vi "SCMP - Externally Triggered Image Acquisition - v3.vi"(0 "FPS":dbl=10.0 format="%.1g", 1 "LCVR Voltages":dbl[][](array[numeric]), 5 "Modulation Cycles":i32=1 min=1 max=30 step=1, 7 "Save to FITS?":bool=TRUE, 9 "Headers In":T12[](array[typedef])=[{"Wavelength (nm)"=530.15, "Exposure (s)"=0.05, "Tuning Delay (ms)"=1000.0, "Beam Type (-1/1)"=1.0, "Tuning Voltages"=[1.111, 2.222, 3.333, 4.444], "Observer"="observer", "Light Shapping Diffuser"=enum."In Beam", "Comment"="", "Data Type"=9, "Mod Cycles"=0, "SCD Calibration Optics"=enum."1 - Polarizer @0, I+Q", "SCD Emission Line Filter"=enum."1-557.6nm", "Cookbook"="", "COMP-S Calibration Wheel"=enum."Dark", "COMP-S Andover Filter Wheel"=enum."530.3nm/HWB 0.34nm (Fe XIV)", "FOV Rotation (deg)"=66.0, "Objective Lens Position (mm)"=0.0, "Occulter size"=0.0, "Time End"=timestamp(3382374145.421875 s since 1904-01-01), "Acc Exposure (s)"=0.0, "Time Stamp Array"=[], "Camera Serial Number"=[], "Camera Temp"=[], "Camera PI (mm)"=[], "Time Start"=timestamp(3382374145.421875 s since 1904-01-01), "Peripherals"={"ILX controler"=FALSE, "Zone temperatures"=FALSE, "Andor"=FALSE, "Andor 2"=FALSE, "PI Stages"=FALSE, "AISAS mechanisms"=FALSE, "AISAS Mech.lvclass"=refnum, "Zone temp ref"=variant, "FWs"=FALSE}, "FITS paths"=[], "Cameras"=enum."Andor", "load preset cbk"=FALSE, "periodic check count"=0, "COMP-S Calibration Wheel 2"=enum."Dark", "Calib"=enum."Dark", "Abso Aperture"=40.0, "Nominal Aperture"=196.0}] {"Nominal Aperture" format="%.1f"; "Abso Aperture" format="%.1f"; "Camera PI (mm)" format="%_3g"; "Acc Exposure (s)" format="%^.3g"; "Occulter size" format="%.2f"; "Objective Lens Position (mm)" min=70.0 max=152.0 format="%.2f"; "FOV Rotation (deg)" format="%.1f"; "Data Type" items=["LIVE", "DARK", "FLAT", "CALI", "OBSE", "ABSO", "AURE", "TARG", "OBJE", "HOLE", "OREX", "THRO", "CHIP"]; "Exposure (s)" format="%^.3g"; "Wavelength (nm)" format="%_6g"}, 11 "error in":errorcluster, 12 "Andor Neo":T13[](array[typedef]) {"Exposure (s)" format="%^.3g"; "Time at Synch" format="%<%H:%M:%S>T"; "Interframe Time" format="%#_3g"; "Frame Readout Time" format="%_3g"; "Row Readout Time" format="%_3g"}) -> (3 "FITS Path Out":path, 6 "Image":u32[][](array[numeric]), 8 "Image Cam2":u32[][](graph), 10 "Headers Out":T2[](array[typedef]) {"Nominal Aperture" format="%.1f"; "Abso Aperture" format="%.1f"; "Camera PI (mm)" format="%_3g"; "Acc Exposure (s)" format="%^.3g"; "Occulter size" format="%.2f"; "Objective Lens Position (mm)" min=70.0 max=152.0 format="%.2f"; "FOV Rotation (deg)" format="%.1f"; "Exposure (s)" format="%^.3g"; "Wavelength (nm)" format="%_6g"}, 13 "FITS Path Out 2":path, 14 "Break":bool, 15 "error out":errorcluster)   [LabVIEW 2014]
doc: "The LL Sequence VI acquires a sequence of images and displays them in an array of image controls using the low-level acquisition VIs. A sequence is appropriate for applications that process multiple images. You can configure a sequence to acquire every frame or to skip a variable number of frames between each image.\n\nTop Level Code Overview\n1) Initialize Camera (Global Shutter, High Well, Low Noise, exposure time, etc.)\n2) Create a buffer set equal in size to the # of trigger pulses (e.g. 100) which is the same as the # of expected images \n3) Start the camera acquisition THEN start the DAQmx task (use merge error cluster to gurantee this)"
uses:
  Camera/Andor Neo Info.ctl
  Controls/run cbk timeout.ctl
  <vilib>/Waveform/WDTOps.llb/WDT Waveform Duration DBL.vi
  <vilib>/DAQmx/write.llb/DAQmx Write (Analog 1D Wfm NChan NSamp).vi
  <vilib>/DAQmx/create/channels.llb/DAQmx Create Channel (AO-Voltage-Basic).vi
  <vilib>/DAQmx/configure/timing.llb/DAQmx Timing (Use Waveform).vi
  Controls/beaning.ctl
  Controls/SCD - Calibration Optics Filter Wheel.ctl
  AISAS/Controls/Diffuser.ctl
  Controls/SCD - FITS Cluster.ctl
  Controls/SCD - EDT - Emission Line Filter Wheel.ctl
  Controls/CoMP-S Controls/Polarization Optics Filter Wheel.ctl
  Controls/CoMP-S Controls/Emission Line Filter Wheel.ctl
  AISAS/Controls/focus.ctl
  AISAS/Mech/AISAS Mech.lvclass
  Controls/peripherals.ctl
  Controls/Cameras select.ctl
  Controls/FITS Data type.ctl
panel:
  out "error dequeue RAM":errorcluster
  out "mod cycles *4":i32=1
  out "error cam dequeue & queue RAM":errorcluster
  out "error dequeue 2":errorcluster
  in  "count 2":i32
  in  "Tab Control":T1(tab)
  out "# elements in RAM queue":i32
  out "Image Acq (s)":dbl(slide)=4151.832132564842
  out "Image display & SSD Saving":i32(slide) scale=0.0..1.0
  in  "user break":bool
  out "Image Cam1 wide":u32[][](graph)
  out "Image Cam1":u32[][](graph)
  out "# images to acquire":i32
  out "Image Acquisition Started":bool
  out "PixelData [U16]":u16[](array[numeric])
  out "ByteData [U8]":u8[](array[numeric])
  in  "image pointers":u64[](array[numeric])
  in  "imageNo":i32
  in  "count":i32
  out "# wavelengths":i32=1
  out "Exposure Get (s)":dbl=0.09 format="%_3p"
  out "# elements in queue":i32
  out "Image Cam":u32[][](graph)
  out "# buffer":i32
  in  "image pointers 2":u64[](array[numeric])
  in  "imageNo 2":i32
  out "# elements in queue 2":i32
  out "# buffer 2":i32
  out "Image transfering":u32(slide) scale=0.0..4.0
  out "Acquisition Estimate (s)":dbl format="%0.2f"
  out "Image Acq":i32(slide) scale=0.0..4.0
  out "Time Start":timestamp=timestamp(3382374145.421875 s since 1904-01-01) format="%<%H:%M:%S%3u\n%x>T"
  out "Time stamp arr":timestamp[](array[timestamp]) format="%<%H:%M:%S%3u>T"
  out "COMP Waveforms":waveform(dbl)[](graph)
  out "SCD Waveforms":waveform(dbl)[](graph)
  out "Time stamp arr 2":timestamp[](array[timestamp]) format="%<%H:%M:%S%3u>T"
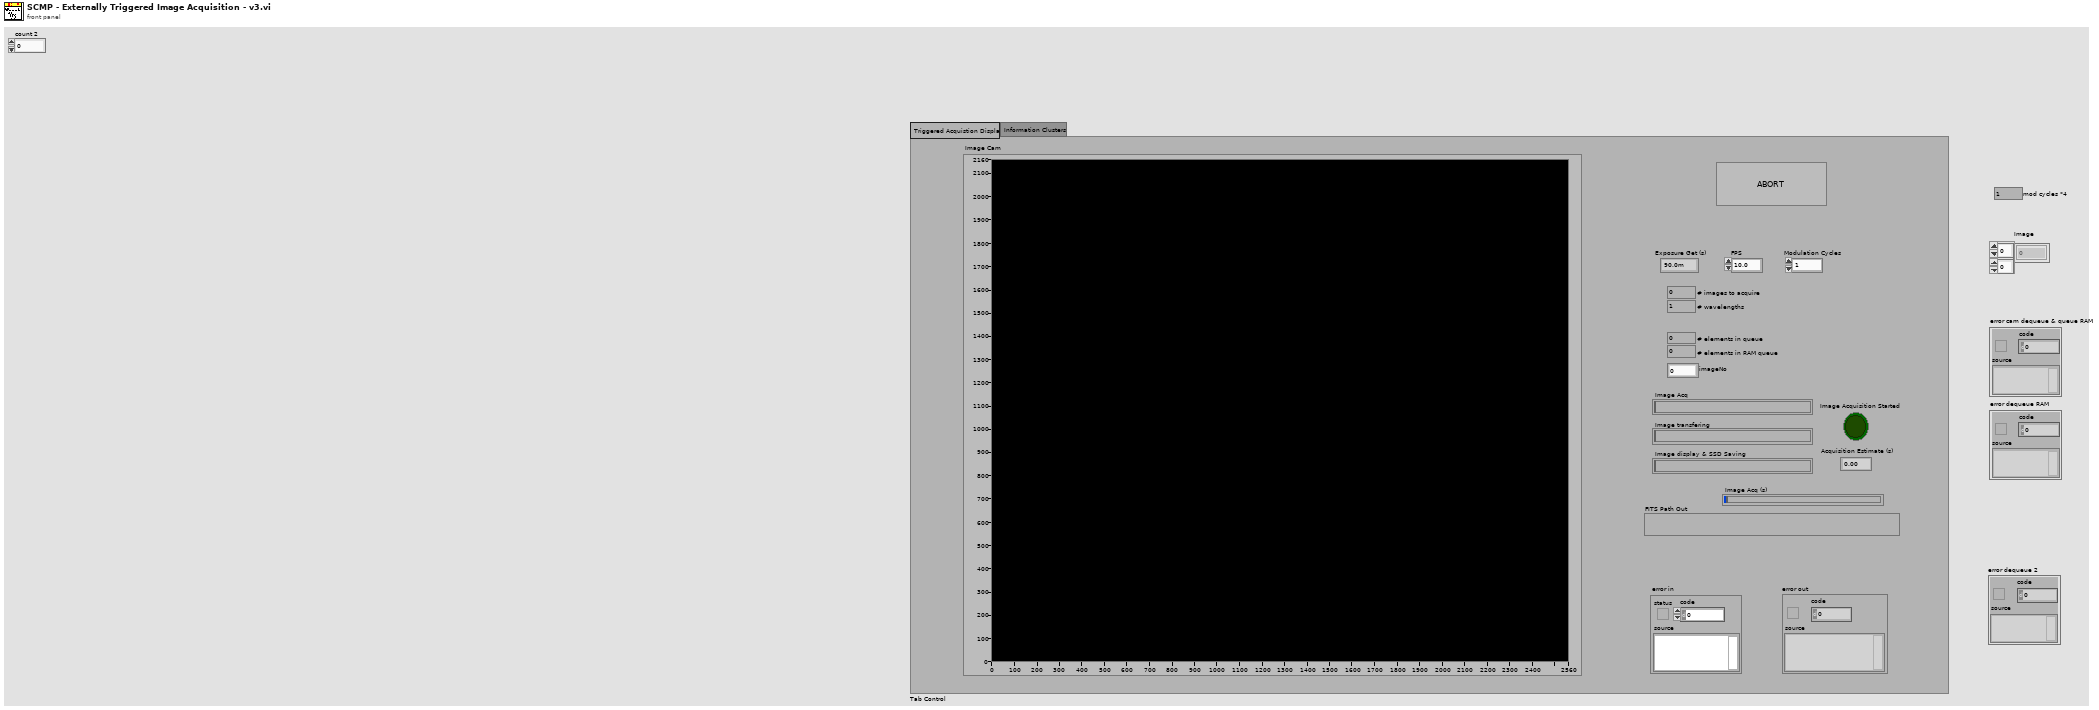
[diagram p1: front panel]
types:
  T1 = enum32{"Triggered Acquistion Display", "Information Clusters"}
  T2 = typedef "SCD - FITS Cluster.ctl" = cluster{"Wavelength (nm)":dbl, "Exposure (s)":dbl, "Tuning Delay (ms)":dbl, "Beam Type (-1/1)":dbl, "Tuning Voltages":dbl[], "Observer":string, "Light Shapping Diffuser":T3, "Comment":string, "Data Type":T4, "Mod Cycles":u16, "SCD Calibration Optics":T5, "SCD Emission Line Filter":T6, "Cookbook":string, "COMP-S Calibration Wheel":T7, "COMP-S Andover Filter Wheel":T8, "FOV Rotation (deg)":dbl, "Objective Lens Position (mm)":T9, "Occulter size":dbl, "Time End":timestamp, "Acc Exposure (s)":dbl, "Time Stamp Array":timestamp[], "Camera Serial Number":string[], "Camera Temp":dbl[], "Camera PI (mm)":dbl[], "Time Start":timestamp, "Peripherals":T10, "FITS paths":path[], "Cameras":T11, "load preset cbk":bool, "periodic check count":i32, "COMP-S Calibration Wheel 2":T7, "Calib":enum16{"Dark", "Flat"}, "Abso Aperture":dbl, "Nominal Aperture":dbl, "Pointer IP":string}
  T3 = typedef "Diffuser.ctl" = enum16{"Out of Beam", "In Beam"}
  T4 = typedef "FITS Data type.ctl" = enum16{"LIVE", "DARK", "FLAT", "CALI", "OBSE", "ABSO", "AURE", "TARG", "OBJE", "HOLE", "OREX", "THRO", "CHIP"}
  T5 = typedef "SCD - Calibration Optics Filter Wheel.ctl" = enum16{"1 - Polarizer @0, I+Q", "2 - Polarizer @90, I-Q", "3 - Polarizer @45, I+U", "4 - Polarizer @135, I-U", "5 - Polarizer @0, Retarder @45, I+V", "6 - Polarizer @0, Retarder @135, I-V", "7 - Dark", "8 - Clear", "9 - N/A"}
  T6 = typedef "SCD - EDT - Emission Line Filter Wheel.ctl" = enum16{"1-557.6nm", "2-587.6nm", "3-589.6nm", "4-630.2nm", "5-656.4nm", "6-849.8nm", "7-854.2nm", "8-866.2nm", "9-1083.0nm"}
  T7 = typedef "Polarization Optics Filter Wheel.ctl" = enum16{"Dark", "Clear", "Exchange Lens", "Polarizer @0, I+Q", "Polarizer @90, I-Q", "Polarizer @45, I+U", "Polarizer @135, I-U", "Polarizer @0, Retarder @45, I+V", "Polarizer @0, Retarder @135, I-V"}
  T8 = typedef "Emission Line Filter Wheel.ctl" = enum16{"530.3nm/HWB 0.34nm (Fe XIV)", "587.6nm/HBW 0.44nm (He I D3)", "637.5nm/HBW 0.53nm (Fe X)", "656.3nm/HBW 0.57nm (H-Alpha)", "789.2nm/HBW 0.85nm (Fe XI)", "854.2nm/HBW 1.01nm (Ca I)", "1074.7nm/HBW 2.34nm (Fe XIII)", "1079.8nm/HBW 1.64nm (Fe XIII)", "1083.0nm/HBW 1.66nm (He I)"}
  T9 = typedef "focus.ctl" = dbl
  T10 = typedef "peripherals.ctl" = cluster{"ILX controler":bool, "Zone temperatures":bool, "Andor":bool, "Andor 2":bool, "PI Stages":bool, "AISAS mechanisms":bool, "AISAS Mech.lvclass":refnum<class "AISAS Mech.lvclass">, "Zone temp ref":variant, "FWs":bool}
  T11 = typedef "Cameras select.ctl" = enum16{"Andor", "GDR"}
  T12 = typedef "SCD - FITS Cluster.ctl" = cluster{"Wavelength (nm)":dbl, "Exposure (s)":dbl, "Tuning Delay (ms)":dbl, "Beam Type (-1/1)":dbl, "Tuning Voltages":dbl[], "Observer":string, "Light Shapping Diffuser":T3, "Comment":string, "Data Type":u16, "Mod Cycles":u16, "SCD Calibration Optics":T5, "SCD Emission Line Filter":T6, "Cookbook":string, "COMP-S Calibration Wheel":T7, "COMP-S Andover Filter Wheel":T8, "FOV Rotation (deg)":dbl, "Objective Lens Position (mm)":T9, "Occulter size":dbl, "Time End":timestamp, "Acc Exposure (s)":dbl, "Time Stamp Array":timestamp[], "Camera Serial Number":string[], "Camera Temp":dbl[], "Camera PI (mm)":dbl[], "Time Start":timestamp, "Peripherals":T10, "FITS paths":path[], "Cameras":T11, "load preset cbk":bool, "periodic check count":i32, "COMP-S Calibration Wheel 2":T7, "Calib":enum16{"Dark", "Flat"}, "Abso Aperture":dbl, "Nominal Aperture":dbl}
  T13 = typedef "Andor Neo Info.ctl" = cluster{"Handle":i32, "Pixel Encoding":string, "AOI Width":i32, "AOI Height":i32, "AOI Stride":i32, "Row Readout Time":dbl, "Frame Readout Time":dbl, "Interframe Time":dbl, "Semaphore":T14, "SerialNumber":string, "Camera Model":string, "Controller ID":string, "Firmware Version":string, "Shutter":string, "BDiv":u8, "Time at Synch":timestamp, "Idx":i32, "PreAmp":string, "Binning":T15, "PixelReadoutRate":string, "Exposure (s)":dbl, "Image Bytes":i64, "Image Pixels":i64, "SpuriousNoiseFilter":bool, "Overlap":bool, "CycleMode":string}
  T14 = typedef "Semaphore RefNum" = refnum<k1>
  T15 = typedef "beaning.ctl" = enum16{"1x1", "2x2", "3x3", "4x4", "8x8"}
  T16 = typedef "run cbk timeout.ctl" = i32
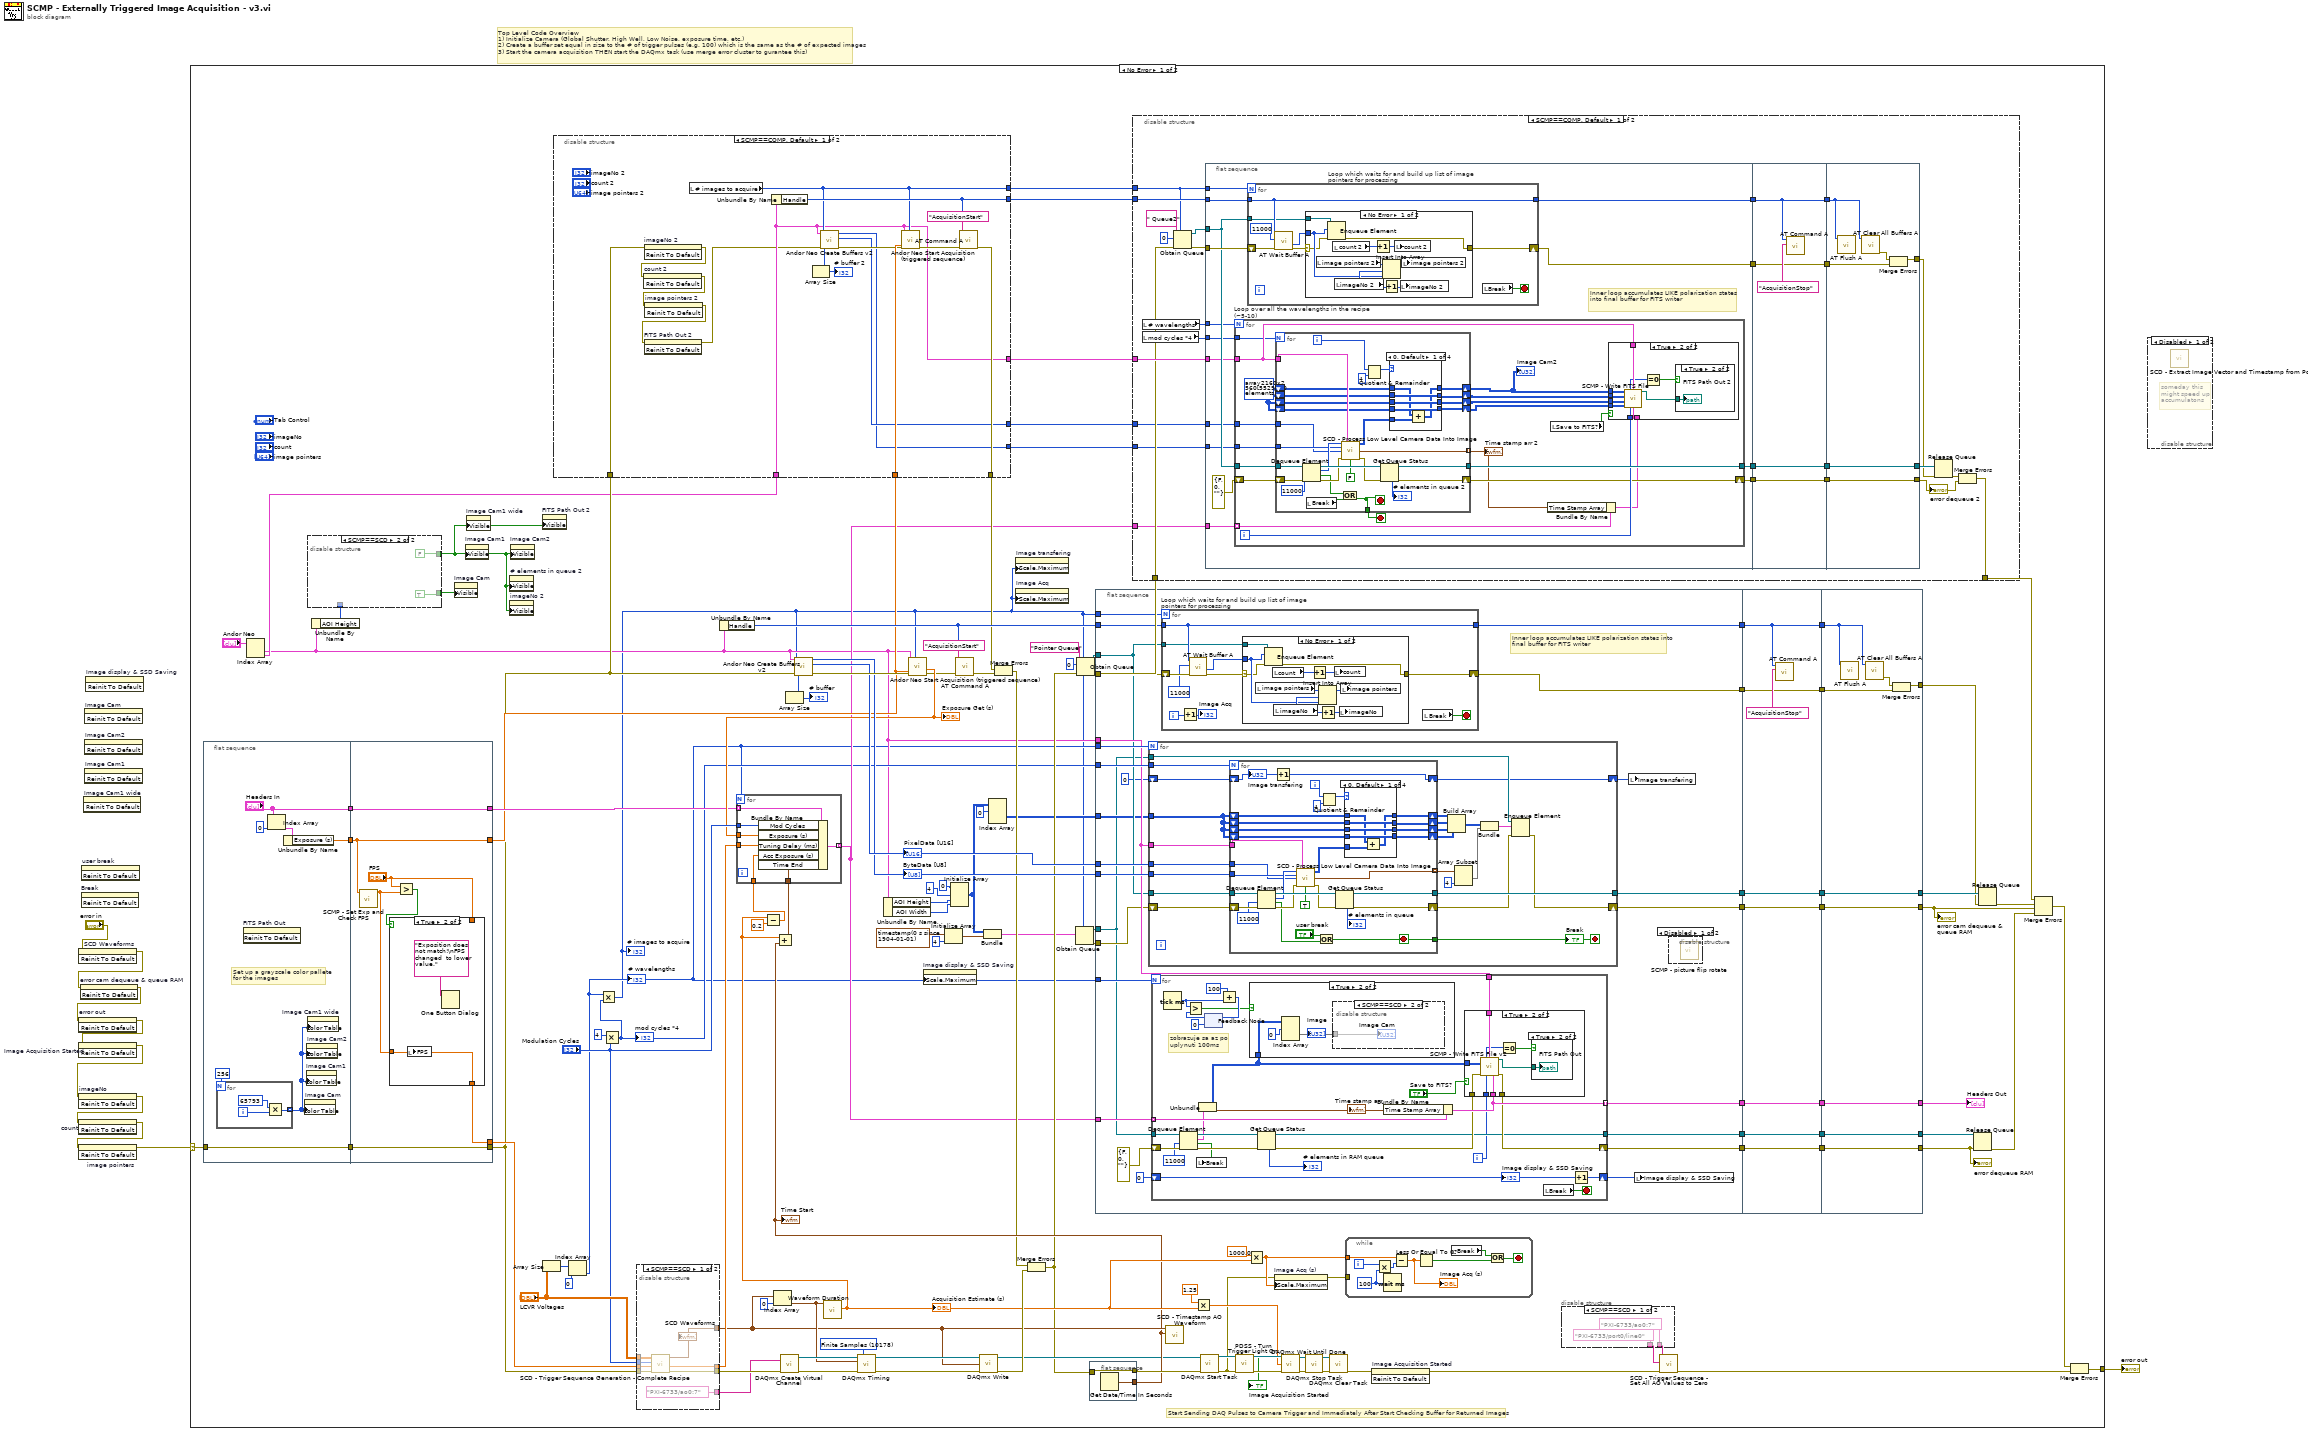
[diagram p0: block diagram]
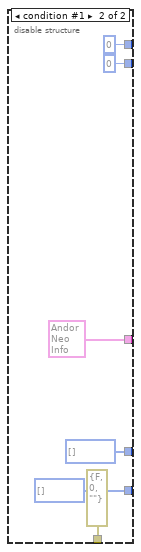
[diagram p3: hidden frame]
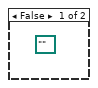
[diagram p4: hidden frame]
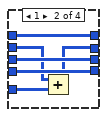
[diagram p6: hidden frame]
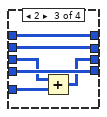
[diagram p7: hidden frame]
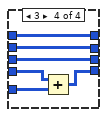
[diagram p8: hidden frame]
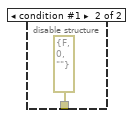
[diagram p10: hidden frame]
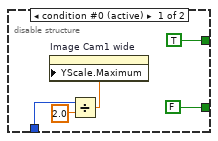
[diagram p12: hidden frame]
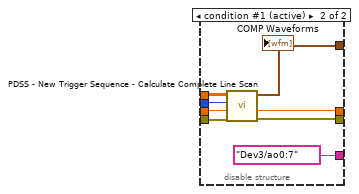
[diagram p13: hidden frame]
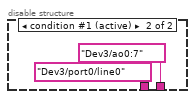
[diagram p14: hidden frame]
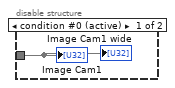
[diagram p17: hidden frame]
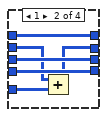
[diagram p20: hidden frame]
diagram:
  # "Top Level Code Overview\n1) Initialize Camera (Global Shutter, High Well, Low Noise, exposure time, etc.)\n2) Create a buffer set equal in size to the # of trigger pulses (e.g. 100) which is the same as the # of expected images \n3) Start the camera acquisition THEN start the DAQmx task (use merge error cluster to gurantee this)"
  n1 = invoke on="SCD Waveforms" class="WFGraph (strict)" method="Reinit To Default"(error in="error in") -> (error out=w3:errorcluster)  [unwired: 2 in, 2 out]
  n2 = invoke on="error cam dequeue & queue RAM" class="Clust (strict)" method="Reinit To Default"(error in=w3) -> (error out=w2:errorcluster)  [unwired: 2 in, 2 out]
  n3 = invoke on="error out" class="Clust (strict)" method="Reinit To Default"(error in=w2) -> (error out=w8:errorcluster)  [unwired: 2 in, 2 out]
  n4 = invoke on="Image Acquisition Started" class="Bool (strict)" method="Reinit To Default"(error in=w8) -> (error out=w4:errorcluster)  [unwired: 2 in, 2 out]
  n5 = invoke on="imageNo" class="DigNum (strict)" method="Reinit To Default"(error in=w4) -> (error out=w7:errorcluster)  [unwired: 2 in, 2 out]
  n6 = invoke on="count" class="DigNum (strict)" method="Reinit To Default"(error in=w7) -> (error out=w6:errorcluster)  [unwired: 2 in, 2 out]
  n7 = invoke on="image pointers" class="Arr (strict)" method="Reinit To Default"(error in=w6) -> (error out=w5:errorcluster)  [unwired: 2 in, 2 out]
  n8 = invoke on="Break" class="Bool (strict)" method="Reinit To Default"() -> ()  [unwired: 3 in, 3 out]
  n9 = invoke on="user break" class="Bool (strict)" method="Reinit To Default"() -> ()  [unwired: 3 in, 3 out]
  n10 = invoke on="Image Cam1 wide" class="IntGraph (strict)" method="Reinit To Default"() -> ()  [unwired: 3 in, 3 out]
  n11 = invoke on="Image Cam" class="IntGraph (strict)" method="Reinit To Default"() -> ()  [unwired: 3 in, 3 out]
  n12 = invoke on="Image Cam2" class="IntGraph (strict)" method="Reinit To Default"() -> ()  [unwired: 3 in, 3 out]
  n13 = invoke on="Image Cam1" class="IntGraph (strict)" method="Reinit To Default"() -> ()  [unwired: 3 in, 3 out]
  n14 = invoke on="Image display & SSD Saving" class="Slide (strict)" method="Reinit To Default"() -> ()  [unwired: 3 in, 3 out]
  n15 = case shown="No Error" w5 {
    selector: w5 -> [w71 w557]
    tunnel: [w102 w557] -> w9
    frame No Error {
      w129 = 10178 items=["Finite Samples"=10178, "Continuous Samples"=10123] ("sample mode")
      # "Start Sending DAQ Pulses to Camera Trigger and Immediately After Start Checking Buffer for Returned Images"
      n16 = flat-sequence {
        tunnel: w71 -> [w321]
        tunnel: [w321] -> w63
        tunnel: ["Headers In"] -> w61
        tunnel: [w316] -> w60
        tunnel: [w332] -> w41
        tunnel: w63 -> [w332]
        tunnel: [w331] -> w62
        tunnel: w61 -> [w331]
        tunnel: [w326] -> w51
        tunnel: w60 -> [w326]
        tunnel: [w329] -> w59
        frame #0 {
          # "Set up a grayscale color pallete for the images"
          n17 = for {
            N: 256 -> [_]
            tunnel: [w324] -> w320 mode=indexing
            i -> [w325]
            n18 = Multiply(x=65793, y=w325) -> (x*y=w324:i32)
          }
          n19 = invoke on="FITS Path Out" class="Path" method="Reinit To Default"() -> ()  [unwired: 3 in, 3 out]
          n20 = Index Array(array="Headers In", index=0) -> (element=w318:T12)
          n21 = Unbundle By Name(w318) -> ("Exposure (s)"=w316:dbl)
          n22 = property on="Image Cam" class="IntGraph (strict)"("Color Table"=w320) -> ()  [unwired: 2 in, 2 out]
          n23 = property on="Image Cam1" class="IntGraph (strict)"("Color Table"=w320) -> ()  [unwired: 2 in, 2 out]
          n24 = property on="Image Cam2" class="IntGraph (strict)"("Color Table"=w320) -> ()  [unwired: 2 in, 2 out]
          n25 = property on="Image Cam1 wide" class="IntGraph (strict)"("Color Table"=w320) -> ()  [unwired: 2 in, 2 out]
        }
        frame #1 {
          n26 = call "SCMP - Set Exp and Check FPS.vi"("Exposure [s]"=w326) -> ("FPS"=w327:dbl)  [unwired: 9 in, 1 out]
          n27 = Greater?(x="FPS", y=w327) -> (0:w330:bool)
          n28 = case shown="True" w330 {
            tunnel: [w333 w334] -> w329
            tunnel: "FPS" -> [w333 _]
            tunnel: w327 -> [_ w334]
            frame False {
            }
            frame True {
              n29 = local write "FPS"(w334) -> ()
              n30 = One Button Dialog(message="Exposition does not match!\nFPS changed  to lower value.") -> ()  [unwired: 1 in, 1 out]
            }
          }
        }
      }
      n31 = Index Array(array="Andor Neo") -> (element #1=w33:T13, element #2=w38:T13)  [unwired: 2 in]
      n32 = Unbundle By Name(w33) -> ("AOI Height"=w79:i32)
      n33 = disable-structure shown="SCMP==SCD" {
        disable-tunnel: w79 -> [w339 _]
        disable-tunnel: [TRUE ("Visible") FALSE ("Visible")] -> w10
        disable-tunnel: [FALSE ("Visible") TRUE ("Visible")] -> w78
        frame condition #0 (active) {
          n34 = Divide(x=w339, y=2.0) -> (x/y=w340:dbl)
          n35 = property on="Image Cam1 wide" class="IntGraph (strict)"("YScale.Maximum"=w340) -> ()  [unwired: 2 in, 2 out]
        }
        frame condition #1 {
        }
      }
      n36 = property on="Image Cam" class="IntGraph (strict)"("Visible"=w78) -> ()  [unwired: 2 in, 2 out]
      n37 = property on="Image Cam1" class="IntGraph (strict)"("Visible"=w10) -> ()  [unwired: 2 in, 2 out]
      n38 = property on="Image Cam1 wide" class="IntGraph (strict)"("Visible"=w10) -> ()  [unwired: 2 in, 2 out]
      n39 = property on="# elements in queue 2" class="DigNum (strict)"("Visible"=w10) -> ()  [unwired: 2 in, 2 out]
      n40 = property on="imageNo 2" class="DigNum (strict)"("Visible"=w10) -> ()  [unwired: 2 in, 2 out]
      n41 = property on="Image Cam2" class="IntGraph (strict)"("Visible"=w10) -> ()  [unwired: 2 in, 2 out]
      n42 = property on="FITS Path Out 2" class="Path"("Visible"=w10) -> ()  [unwired: 2 in, 2 out]
      n43 = Array Size(array="LCVR Voltages") -> (size(s)=w112:i32[])
      n44 = disable-structure shown="SCMP==COMP, Default" {
        disable-tunnel: w51 -> [w154 _]
        disable-tunnel: [w153 errorcluster {"status"=FALSE, "code"=0, "source"=""} ("error out")] -> w48
        disable-tunnel: [w147 0 ("Handle")] -> w45
        disable-tunnel: [w146 i64[] [] ("PixelData")] -> w44
        disable-tunnel: [w145 u8[] [] ("ByteData")] -> w43
        disable-tunnel: [w144 0 ("# images to acquire")] -> w42
        disable-tunnel: w41 -> [w140 _]
        disable-tunnel: [w143 T13 {"Handle"=0, "Pixel Encoding"="", "AOI Width"=0, "AOI Height"=0, "AOI Stride"=0, "Row Readout Time"=0.0, "Frame Readout Time"=0.0, "Interframe Time"=0.0, "Semaphore"=refnum, "SerialNumber"="", "Camera Model"="", "Controller ID"="", "Firmware Version"="", "Shutter"="Global", "BDiv"=1, "Time at Synch"=timestamp(3029526000.379448 s since 1904-01-01), "Idx"=0, "PreAmp"="", "Binning"=enum."1x1", "PixelReadoutRate"="", "Exposure (s)"=0.05, "Image Bytes"=0, "Image Pixels"=0, "SpuriousNoiseFilter"=FALSE, "Overlap"=FALSE, "CycleMode"=""} ("Neo Info")] -> w39
        disable-tunnel: w38 -> [w143 _]
        frame condition #0 (active) {
          n45 = invoke on="imageNo 2" class="DigNum (strict)" method="Reinit To Default"(error in=w140) -> (error out=w142:errorcluster)  [unwired: 2 in, 2 out]
          n46 = invoke on="count 2" class="DigNum (strict)" method="Reinit To Default"(error in=w142) -> (error out=w141:errorcluster)  [unwired: 2 in, 2 out]
          n47 = invoke on="image pointers 2" class="Arr (strict)" method="Reinit To Default"(error in=w141) -> (error out=w139:errorcluster)  [unwired: 2 in, 2 out]
          n48 = invoke on="FITS Path Out 2" class="Path" method="Reinit To Default"(error in=w139) -> (error out=w138:errorcluster)  [unwired: 2 in, 2 out]
          n49 = local read "# images to acquire"() -> (w144:i32)
          n50 = Unbundle By Name(w143) -> ("Handle"=w147:i32)
          n51 = call "Andor Neo Create Buffers v2.vi"("error in"=w138, "Number of Images"=w144, "Camera Info"=w143) -> ("error out"=w151:errorcluster, "PixelData"=w146:i64[], "ByteData"=w145:u8[], "# of Andor buffers"=w149:i32)  [unwired: 4 in, 1 out]
          n52 = Array Size(array=w149) -> (size(s)=→"# buffer 2":i32)
          n53 = call "Andor Neo Start Acquisition (triggered sequence).vi"("Exposure Set (s)"=w154, "error in"=w151, "Frames"=w144, "Camera Info"=w143) -> ("error out"=w150:errorcluster)  [unwired: 6 in, 1 out]
          n54 = call <userlib>:"AT Command A.vi"("error in (no error)"=w150, "Feature"="AcquisitionStart" ("Command"), "Handle"=w147) -> ("error out"=w153:errorcluster)  [unwired: 7 in, 1 out]
        }
        frame condition #1 {
        }
      }
      n55 = Index Array(array=w112, index=0) -> (element=w12:i32)
      "# wavelengths" <- w12
      n56 = Multiply(x=4 ("value"), y="Modulation Cycles") -> (x*y=w40:i32)
      "mod cycles *4" <- w40
      n57 = Multiply(x=w12, y=w40) -> (x*y=w11:i32)
      "# images to acquire" <- w11
      n58 = disable-structure shown="SCMP==SCD" {
        disable-tunnel: [w350 w354] -> w120
        disable-tunnel: "LCVR Voltages" -> [w349 w358]
        disable-tunnel: [w344 w352] -> w84
        disable-tunnel: w59 -> [w348 w356]
        disable-tunnel: w41 -> [w347 w355]
        disable-tunnel: [w346 w353] -> w87
        disable-tunnel: "Modulation Cycles" -> [w345 w357]
        disable-tunnel: [tag "PXI-6733/ao0:7" ("physical channels") tag "Dev3/ao0:7" ("physical channels")] -> w57
        frame condition #0 {
          n59 = call "SCD - Trigger Sequence Generation - Complete Recipe.vi"("error in"=w347, "FPS"=w348, "Modulation Cycles\nAt Each Wavelength"=w345, "LCVR Voltages"=w349) -> ("error out"=w350:errorcluster, "LCVR Relaxtion Time"=w346:dbl, "SCD Waveforms (Graph)"=w344:waveform(dbl)[])  [unwired: 5 in]
          "SCD Waveforms" <- w344
        }
        frame condition #1 (active) {
          n60 = call "PDSS - New Trigger Sequence - Calculate Complete Line Scan.vi"("error in"=w355, "FPS"=w356, "Modulation Cycles\nAt Each Wavelength"=w357, "LCVR Voltages"=w358) -> ("error out"=w354:errorcluster, "LCVR Relaxtion Time"=w353:dbl, "AO Graph"=w352:waveform(dbl)[])  [unwired: 5 in]
          "COMP Waveforms" <- w352
        }
      }
      n61 = Unbundle By Name(w33) -> ("Handle"=w53:i32)
      n62 = Index Array(array=w84, index=0) -> (element=w117:waveform(dbl))
      n63 = call-poly <vilib>:"DAQmx Create Virtual Channel.vi"("physical channels"=w57, "error in"=w120) -> ("task out"=w127:refnum<k21>, "error out"=w128:errorcluster)  [unwired: 12 in]
      n64 = call "Andor Neo Create Buffers v2.vi"("error in"=w41, "Number of Images"=w11, "Camera Info"=w33) -> ("error out"=w101:errorcluster, "PixelData"=w97:i64[], "ByteData"=w96:u8[], "# of Andor buffers"=w70:i32)  [unwired: 4 in, 1 out]
      "ByteData [U8]" <- w96
      "PixelData [U16]" <- w97
      n65 = Array Size(array=w70) -> (size(s)=→"# buffer":i32)
      n66 = call-poly <vilib>:"Waveform Duration.vi"("waveform in"=w117) -> ("duration"=w73:dbl)  [unwired: 8 in, 2 out]
      "Acquisition Estimate (s)" <- w73
      n67 = Subtract(x=w73, y=0.2) -> (x-y=w72:dbl)
      n68 = Add(x=w73, y=w58) -> (x+y=w77:timestamp)
      n69 = call-poly <vilib>:"DAQmx Timing.vi"("task/channels in"=w127, "sample mode"=w129, "waveform"=w117, "error in"=w128) -> ("task out"=w118:refnum<k21>, "error out"=w119:errorcluster)  [unwired: 10 in]
      n70 = Unbundle By Name(w33) -> ("AOI Height"=w15:i32, "AOI Width"=w14:i32)
      n71 = call "Andor Neo Start Acquisition (triggered sequence).vi"("Exposure Set (s)"=w51, "error in"=w101, "Frames"=w11, "Camera Info"=w33) -> ("error out"=w75:errorcluster, "Exposure Get (s)"=w76:dbl)  [unwired: 6 in]
      "Exposure Get (s)" <- w76
      n72 = for {
        N: w12 -> [_]
        tunnel: [w369] -> w47 mode=indexing
        tunnel: w76 -> [w368]
        tunnel: w62 -> [w367] mode=indexing
        tunnel: w87 -> [w366]
        tunnel: "Modulation Cycles" -> [w365]
        tunnel: w72 -> [w364]
        tunnel: w77 -> [w363]
        n73 = Bundle By Name(cluster=w367, "Mod Cycles"=w365, "Exposure (s)"=w368, "Tuning Delay (ms)"=w366, "Acc Exposure (s)"=w364, "Time End"=w363) -> (w369:T12)
      }
      n74 = property on="Image display & SSD Saving" class="Slide (strict)"("Scale.Maximum"=w12) -> ()  [unwired: 2 in, 2 out]
      n75 = Initialize Array(timestamp(0 s since 1904-01-01) ("Timestamp"), 4 ("dimension size")) -> (w27:timestamp[])
      n76 = Initialize Array(u32 0, 4 ("dimension size"), w15, w14) -> (w18:u32[][][])
      n77 = call <userlib>:"AT Command A.vi"("error in (no error)"=w75, "Feature"="AcquisitionStart" ("Command"), "Handle"=w53) -> ("error out"=w100:errorcluster)  [unwired: 7 in, 1 out]
      n78 = call-poly <vilib>:"DAQmx Write.vi"("task/channels in"=w118, "data"=w84, "error in"=w119) -> ("task out"=w52:refnum<k21>, "error out"=w104:errorcluster)  [unwired: 10 in, 1 out]
      n79 = Bundle(w18, w27) -> (w13:cluster{u32[][][], timestamp[]})  [unwired: 1 in]
      n80 = Index Array(array=w18, index (dim 0)=0 ("disabled index (col)")) -> (element=w17:u32[][])  [unwired: 2 in]
      n81 = Merge Errors(w48, w100) -> (w49:errorcluster)
      n82 = property on="Image transfering" class="Slide (strict)"("Scale.Maximum"=w11) -> ()  [unwired: 2 in, 2 out]
      n83 = property on="Image Acq" class="Slide (strict)"("Scale.Maximum"=w11) -> ()  [unwired: 2 in, 2 out]
      n84 = Merge Errors(w49, w104) -> (w50:errorcluster)
      n85 = Obtain Queue(max queue size (-1, unlimited)=w11, element data type=w13) -> (queue out=w30:refnum<queue>, error out=w31:errorcluster)  [unwired: 3 in, 1 out]
      n86 = Obtain Queue(max queue size (-1, unlimited)=w11, name (unnamed)="Pointer Queue", element data type=u64 0 ("Output buffer"), error in (no error)=w50) -> (queue out=w93:refnum<queue>, error out=w94:errorcluster)  [unwired: 1 in, 1 out]
      n87 = flat-sequence {
        tunnel: [w371] -> w99
        tunnel: w50 -> [w371]
        tunnel: [w370] -> w58
        frame #0 {
          n88 = Get Date/Time In Seconds() -> (seconds since 1Jan1904=w370:timestamp)
        }
      }
      n89 = flat-sequence {
        tunnel: w94 -> [w397]
        tunnel: w11 -> [w389]
        tunnel: w53 -> [w396]
        tunnel: [w395] -> w106
        tunnel: [w387] -> w105
        tunnel: w33 -> [w385]
        tunnel: w47 -> [w391]
        tunnel: [w390] -> w98
        tunnel: w97 -> [w392]
        tunnel: w96 -> [w394]
        tunnel: w93 -> [w380]
        tunnel: [w393] -> w91
        tunnel: w12 -> [w386]
        tunnel: w40 -> [w388]
        tunnel: [w384] -> w82
        tunnel: w31 -> [w383]
        tunnel: w30 -> [w376]
        tunnel: w12 -> [w381]
        tunnel: [w379] -> w26
        tunnel: [w378] -> w24
        tunnel: w17 -> [w377]
        tunnel: w106 -> [w543]
        tunnel: w105 -> [w542]
        tunnel: w98 -> [w546]
        tunnel: w91 -> [w545]
        tunnel: w82 -> [w544]
        tunnel: [w543] -> w68
        tunnel: [w546] -> w67
        tunnel: [w545] -> w66
        tunnel: [w544] -> w65
        tunnel: [w542] -> w64
        tunnel: w26 -> [w541]
        tunnel: [w541] -> w25
        tunnel: w24 -> [w540]
        tunnel: [w540] -> w23
        tunnel: [w554] -> w55
        tunnel: [w555] -> w90
        tunnel: [w556] -> w88
        tunnel: [w553] -> w89
        tunnel: w68 -> [w551]
        tunnel: w67 -> [w556]
        tunnel: w66 -> [w555]
        tunnel: w65 -> [w554]
        tunnel: w64 -> [w552]
        tunnel: w25 -> [w549]
        tunnel: [w549] -> w20
        tunnel: w23 -> [w548]
        tunnel: [w548] -> w22
        frame #0 {
          # "Inner loop accumulates LIKE polarization states into final buffer for FITS writer"
          n90 = for {
            N: w386 -> [_]
            tunnel: w394 -> [w461]
            tunnel: w392 -> [w459]
            tunnel: w385 -> [w458]
            tunnel: w388 -> [w457]
            shift-right: [w449] -> w384
            shift-left: w383 -> [w456]
            tunnel: w380 -> [w462]
            tunnel: [w460] -> w393
            tunnel: w376 -> [w448]
            tunnel: w377 -> [w442]
            shift-right: [w440] -> w372
            shift-left: u32 0 ("Image transfering") -> [w441]
            stop <- w455 stop-if-true
            n91 = for {
              N: w457 -> [_]
              tunnel: w462 -> [w494]
              tunnel: w461 -> [w491]
              tunnel: [w477] -> w460
              tunnel: w459 -> [w490]
              tunnel: w458 -> [w489]
              shift-right: [w482] -> w454
              shift-left: w442 -> [w483]
              shift-right: [w481] -> w453
              shift-left: w442 -> [w484]
              shift-right: [w480] -> w452
              shift-left: w442 -> [w485]
              shift-right: [w479] -> w451
              shift-left: w442 -> [w486]
              shift-right: [w473] -> w450
              shift-left: w456 -> [w471]
              tunnel: [w470] -> w446 mode=indexing
              tunnel: [w466] -> w455
              shift-right: [w463] -> w440
              shift-left: w441 -> [w464]
              i -> [w472]
              stop <- w466 stop-if-true
              n92 = Dequeue Element(queue=w494, timeout in ms (-1)=T16 11000 ("timeout for deque loop"), error in (no error)=w471) -> (queue out=w493:refnum<queue>, element=w492:u64, timed out?=w468:bool, error out=w475:errorcluster)
              n93 = Increment(x=w464) -> (x+1=w463:u32)
              n94 = call "SCD - Process Low Level Camera Data Into Image.vi"("Pointer In"=w492, "Neo Info"=w489, "ByteData (U8)"=w491, "PixelData (U16)"=w490, "error in (no error)"=w475, "scmp demo pic"=TRUE) -> ("Image (I32)"=w478:u32[][], "Timestamp"=w470:timestamp, "error out"=w474:errorcluster)  [unwired: 7 in]
              n95 = Or(x=w468, y="user break") -> (x .or. y?=w466:bool)
              n96 = Quotient & Remainder(x=w472, y=4) -> (x-y*floor(x/y)=w487:i32)  [unwired: 1 out]
              n97 = Get Queue Status(queue=w493, error in (no error)=w474) -> (queue out=w477:refnum<queue>, error out=w473:errorcluster, # elements in queue=→"# elements in queue":i32)  [unwired: 1 in, 5 out]
              n98 = case shown="0, Default" w487 {
                tunnel: w486 -> [w498 w505 w511 w514]
                tunnel: w485 -> [w499 w506 w508 w517]
                tunnel: w484 -> [w500 w502 w512 w518]
                tunnel: w483 -> [w496 w503 w509 w515]
                tunnel: [w495 w503 w509 w515] -> w482
                tunnel: [w500 w501 w512 w518] -> w481
                tunnel: [w499 w506 w507 w517] -> w480
                tunnel: [w498 w505 w511 w513] -> w479
                tunnel: w478 -> [w497 w504 w510 w516]
                frame 0, Default {
                  n99 = Add(x=w496, y=w497) -> (x+y=w495:u32[][])
                }
                frame 1 {
                  n100 = Add(x=w502, y=w504) -> (x+y=w501:u32[][])
                }
                frame 2 {
                  n101 = Add(x=w508, y=w510) -> (x+y=w507:u32[][])
                }
                frame 3 {
                  n102 = Add(x=w514, y=w516) -> (x+y=w513:u32[][])
                }
              }
              "Image transfering" <- w464
            }
            "Break" <- w455
            n103 = Build Array(w454, w453, w452, w451) -> (w444:u32[][][])
            n104 = Array Subset(array=w446, length=4) -> (w443:timestamp[])  [unwired: 1 in]
            n105 = Bundle(w444, w443) -> (w445:cluster{u32[][][], timestamp[]})  [unwired: 1 in]
            n106 = Enqueue Element(queue=w448, element=w445, error in (no error)=w450) -> (error out=w449:errorcluster)  [unwired: 1 in, 2 out]
          }
          n107 = for {
            N: w381 -> [_]
            tunnel: w391 -> [w424] mode=indexing
            tunnel: [w423] -> w390 mode=indexing
            tunnel: w385 -> [w422]
            shift-right: [w420] -> w379
            shift-left: errorcluster {"status"=FALSE, "code"=0, "source"=""} ("error out") -> [w418]
            tunnel: w376 -> [w415]
            tunnel: [w413] -> w378
            shift-right: [w399] -> w373
            shift-left: 0 -> [w398]
            i -> [w400]
            stop <- w419 stop-if-true
            # "zobrazuje sa az po uplynuti 100ms"
            n108 = Tick Count (ms)() -> (millisecond timer value=w404:u32)
            n109 = Dequeue Element(queue=w415, timeout in ms (-1)=T16 11000, error in (no error)=w418) -> (queue out=w414:refnum<queue>, element=w409:cluster{u32[][][], timestamp[]}, timed out?=w412:bool, error out=w417:errorcluster)
            n110 = local write "Break"(w412) -> ()
            n111 = Unbundle(w409) -> (w407:u32[][][], w411:timestamp[])
            "Time stamp arr" <- w411
            n112 = feedback #1(u32 0) -> (w405:u32)
            n113 = Greater?(x=w404, y=w405) -> (0:w401:bool)
            n114 = Add(x=u32 100 ("y"), y=w404) -> (x+y=w406:u32)
            n115 = feedback-in #1(w406) -> ()
            n116 = case shown="True" w401 {
              tunnel: w407 -> [_ w425]
              frame False {
              }
              frame True {
                n117 = Index Array(array=w425, index (dim 0)=0 ("disabled index (col)")) -> (element=w427:u32[][])  [unwired: 2 in]
                "Image" <- w427
                n118 = disable-structure shown="SCMP==SCD" {
                  disable-tunnel: w427 -> [w428 w429]
                  frame condition #0 (active) {
                    "Image Cam1" <- w428
                    "Image Cam1 wide" <- w428
                  }
                  frame condition #1 {
                    "Image Cam" <- w429
                  }
                }
              }
            }
            n119 = Get Queue Status(queue=w414, error in (no error)=w417) -> (queue out=w413:refnum<queue>, error out=w416:errorcluster, # elements in queue=→"# elements in RAM queue":i32)  [unwired: 1 in, 5 out]
            n120 = Bundle By Name(cluster=w424, "Time Stamp Array"=w411) -> (w423:T12)
            n121 = case shown="True" "Save to FITS?" {
              tunnel: w423 -> [_ w438]
              tunnel: w422 -> [_ w437]
              tunnel: w400 -> [_ w436]
              tunnel: [w430 w433] -> w420
              tunnel: w416 -> [w430 w432]
              tunnel: w407 -> [_ w431]
              frame False {
              }
              frame True {
                n122 = call "SCMP - Write FITS File v2.vi"("FITS Header"=w438, "Andor"=w437, "Data"=w431, "error in"=w432, "Image #"=w436) -> ("FITS Path Out"=w434:path, "error out"=w433:errorcluster)  [unwired: 8 in, 1 out]
                n123 = Equal To 0?(x=w436) -> (x = 0?=w435:bool)
                n124 = case shown="True" w435 {
                  tunnel: w434 -> [_ w439]
                  frame False {
                  }
                  frame True {
                    "FITS Path Out" <- w439
                  }
                }
              }
            }
            n125 = local read "Break"() -> (w419:bool)
            n126 = Increment(x=w398) -> (x+1=w399:i32)
            "Image display & SSD Saving" <- w398
          }
          n127 = for "Loop which waits for and build up list of image pointers for processing" {
            N: w389 -> [_]
            tunnel: w396 -> [w526]
            tunnel: [w526] -> w395
            tunnel: w380 -> [w524]
            shift-right: [w523] -> w387
            shift-left: w397 -> [w528]
            i -> [w520]
            stop <- w522 stop-if-true
            n128 = Increment(x=w520) -> (x+1=→"Image Acq":i32)
            n129 = call <userlib>:"AT Wait Buffer A.vi"("error in (no error)"=w528, "Timeout"=T16 11000 ("timeout for deque loop"), "Handle"=w526) -> ("error out"=w525:errorcluster, "Output buffer"=w527:u64)  [unwired: 5 in, 2 out]
            n130 = case shown="No Error" w525 {
              selector: w525 -> [w530 w539]
              tunnel: w527 -> [w532 _]
              tunnel: [w529 w539] -> w523
              tunnel: w524 -> [w531 _]
              frame No Error {
                n131 = local read "image pointers"() -> (w536:u64[])
                n132 = Enqueue Element(queue=w531, element=w532, error in (no error)=w530) -> (error out=w529:errorcluster)  [unwired: 1 in, 2 out]
                n133 = local read "count"() -> (w538:i32)
                n134 = local read "imageNo"() -> (w533:i32)
                n135 = Increment(x=w538) -> (x+1=w537:i32)
                n136 = Insert Into Array(array=w536, index=w533, new element=w532) -> (w535:u64[])
                n137 = Increment(x=w533) -> (x+1=w534:i32)
                n138 = local write "count"(w537) -> ()
                n139 = local write "imageNo"(w534) -> ()
                n140 = local write "image pointers"(w535) -> ()
              }
              frame Error {
              }
            }
            n141 = local read "Break"() -> (w522:bool)
          }
          n142 = local write "Image transfering"(w372) -> ()
          n143 = local write "Image display & SSD Saving"(w373) -> ()
          n144 = disable-structure shown="Disabled" {
            frame Disabled {
              n145 = call "SCMP - picture flip rotate.vi"() -> ()  [unwired: 8 in, 4 out]
            }
            frame Enabled {
            }
          }
        }
        frame #1 {
          n146 = call <userlib>:"AT Command A.vi"("Feature"="AcquisitionStop" ("Command"), "Handle"=w543) -> ()  [unwired: 8 in, 2 out]
        }
        frame #2 {
          n147 = call <userlib>:"AT Flush A.vi"("Handle"=w551) -> ()  [unwired: 9 in, 2 out]
          n148 = call <userlib>:"AT Clear All Buffers A.vi"("Handle"=w551) -> ("error out"=w550:errorcluster)  [unwired: 9 in, 1 out]
          n149 = Merge Errors(w550, w552) -> (w553:errorcluster)
        }
      }
      n150 = disable-structure shown="SCMP==COMP, Default" {
        disable-tunnel: w39 -> [w178 _]
        disable-tunnel: w50 -> [w177 _]
        disable-tunnel: w47 -> [w176 _]
        disable-tunnel: [w175 errorcluster {"status"=FALSE, "code"=0, "source"=""} ("error IO")] -> w46
        disable-tunnel: w45 -> [w172 _]
        disable-tunnel: w44 -> [w171 _]
        disable-tunnel: w43 -> [w170 _]
        disable-tunnel: w42 -> [w167 _]
        frame condition #0 (active) {
          n151 = local read "# wavelengths"() -> (w166:i32)
          n152 = local read "mod cycles *4"() -> (w161:i32)
          n153 = Obtain Queue(max queue size (-1, unlimited)=w167, name (unnamed)=" Queue2", element data type=u64 0 ("Output buffer"), error in (no error)=w177) -> (queue out=w169:refnum<queue>, error out=w168:errorcluster)  [unwired: 1 in, 1 out]
          n154 = flat-sequence {
            tunnel: w168 -> [w201]
            tunnel: w172 -> [w200]
            tunnel: [w199] -> w186
            tunnel: [w190] -> w185
            tunnel: w178 -> [w194]
            tunnel: w171 -> [w195]
            tunnel: w170 -> [w197]
            tunnel: w169 -> [w198]
            tunnel: [w196] -> w184
            tunnel: w161 -> [w192]
            tunnel: [w193] -> w183
            tunnel: w167 -> [w189]
            tunnel: w176 -> [w188]
            tunnel: w166 -> [w187]
            tunnel: w186 -> [w305]
            tunnel: w185 -> [w304]
            tunnel: w184 -> [w307]
            tunnel: w183 -> [w306]
            tunnel: [w305] -> w182
            tunnel: [w307] -> w181
            tunnel: [w306] -> w180
            tunnel: [w304] -> w179
            tunnel: [w314] -> w163
            tunnel: [w313] -> w162
            tunnel: w182 -> [w311]
            tunnel: w181 -> [w309]
            tunnel: w180 -> [w314]
            tunnel: w179 -> [w312]
            tunnel: [w309] -> w164
            frame #0 {
              # "Inner loop accumulates LIKE polarization states into final buffer for FITS writer"
              n155 = for "Loop over all the wavelengths in the recipe (~5-10)" {
                N: w187 -> [_]
                tunnel: w198 -> [w220]
                tunnel: w197 -> [w219]
                tunnel: [w218] -> w196
                tunnel: w195 -> [w217]
                tunnel: w194 -> [w215]
                tunnel: w192 -> [w214]
                shift-right: [w212] -> w193
                shift-left: errorcluster {"status"=FALSE, "code"=0, "source"=""} ("error out") -> [w211]
                tunnel: w188 -> [w207] mode=indexing
                i -> [w213]
                stop <- w210 stop-if-true
                w216 = u32[][] array2160x2560[5529600 elements] ("2560x2160 Initialized Array")
                n156 = for {
                  N: w214 -> [_]
                  tunnel: w220 -> [w260]
                  tunnel: w219 -> [w257]
                  tunnel: [w243] -> w218
                  tunnel: w217 -> [w256]
                  tunnel: w215 -> [w255]
                  shift-right: [w248] -> w205
                  shift-left: w216 -> [w249]
                  shift-right: [w247] -> w204
                  shift-left: w216 -> [w250]
                  shift-right: [w246] -> w203
                  shift-left: w216 -> [w251]
                  shift-right: [w245] -> w202
                  shift-left: w216 -> [w252]
                  shift-right: [w238] -> w212
                  shift-left: w211 -> [w236]
                  tunnel: [w233] -> w210
                  tunnel: [w235] -> w208 mode=indexing
                  i -> [w237]
                  stop <- w233 stop-if-true
                  n157 = Dequeue Element(queue=w260, timeout in ms (-1)=11000, error in (no error)=w236) -> (queue out=w259:refnum<queue>, element=w258:u64, timed out?=w232:bool, error out=w240:errorcluster)
                  n158 = local read "Break"() -> (w231:bool)
                  n159 = Or(x=w232, y=w231) -> (x .or. y?=w233:bool)
                  n160 = call "SCD - Process Low Level Camera Data Into Image.vi"("Pointer In"=w258, "Neo Info"=w255, "ByteData (U8)"=w257, "PixelData (U16)"=w256, "error in (no error)"=w240, "scmp demo pic"=FALSE) -> ("Image (I32)"=w244:u32[][], "Timestamp"=w235:timestamp, "error out"=w239:errorcluster)  [unwired: 7 in]
                  n161 = Quotient & Remainder(x=w237, y=4) -> (x-y*floor(x/y)=w253:i32)  [unwired: 1 out]
                  n162 = Get Queue Status(queue=w259, error in (no error)=w239) -> (queue out=w243:refnum<queue>, error out=w238:errorcluster, # elements in queue=→"# elements in queue 2":i32)  [unwired: 1 in, 5 out]
                  n163 = case shown="0, Default" w253 {
                    tunnel: w252 -> [w264 w271 w277 w280]
                    tunnel: w251 -> [w265 w272 w274 w283]
                    tunnel: w250 -> [w266 w268 w278 w284]
                    tunnel: w249 -> [w262 w269 w275 w281]
                    tunnel: [w261 w269 w275 w281] -> w248
                    tunnel: [w266 w267 w278 w284] -> w247
                    tunnel: [w265 w272 w273 w283] -> w246
                    tunnel: [w264 w271 w277 w279] -> w245
                    tunnel: w244 -> [w263 w270 w276 w282]
                    frame 0, Default {
                      n164 = Add(x=w262, y=w263) -> (x+y=w261:u32[][])
                    }
                    frame 1 {
                      n165 = Add(x=w268, y=w270) -> (x+y=w267:u32[][])
                    }
                    frame 2 {
                      n166 = Add(x=w274, y=w276) -> (x+y=w273:u32[][])
                    }
                    frame 3 {
                      n167 = Add(x=w280, y=w282) -> (x+y=w279:u32[][])
                    }
                  }
                }
                "Time stamp arr 2" <- w208
                "Image Cam2" <- w205
                n168 = Bundle By Name(cluster=w207, "Time Stamp Array"=w208) -> (w209:T12)
                n169 = local read "Save to FITS?"() -> (w206:bool)
                n170 = case shown="True" w206 {
                  tunnel: w204 -> [_ w227]
                  tunnel: w203 -> [_ w228]
                  tunnel: w202 -> [_ w229]
                  tunnel: w209 -> [_ w225]
                  tunnel: w205 -> [_ w226]
                  tunnel: w215 -> [_ w224]
                  tunnel: w213 -> [_ w223]
                  frame False {
                    (unwired) path "" ("FITS Path Out")
                  }
                  frame True {
                    n171 = call "SCMP - Write FITS File.vi"("A"=w226, "FITS Header"=w225, "Neo Info"=w224, "B"=w227, "C"=w228, "D"=w229, "Image #"=w223) -> ("FITS Path Out"=w222:path)  [unwired: 6 in, 2 out]
                    n172 = Equal To 0?(x=w223) -> (x = 0?=w221:bool)
                    n173 = case shown="True" w221 {
                      tunnel: w222 -> [_ w230]
                      frame False {
                      }
                      frame True {
                        "FITS Path Out 2" <- w230
                      }
                    }
                  }
                }
              }
              n174 = for "Loop which waits for and build up list of image pointers for processing" {
                N: w189 -> [_]
                tunnel: w200 -> [w289]
                tunnel: [w289] -> w199
                tunnel: w198 -> [w287]
                shift-right: [w286] -> w190
                shift-left: w201 -> [w291]
                stop <- w285 stop-if-true
                n175 = call <userlib>:"AT Wait Buffer A.vi"("error in (no error)"=w291, "Timeout"=u32 11000, "Handle"=w289) -> ("error out"=w288:errorcluster, "Output buffer"=w290:u64)  [unwired: 5 in, 2 out]
                n176 = case shown="No Error" w288 {
                  selector: w288 -> [w294 w303]
                  tunnel: w290 -> [w296 _]
                  tunnel: [w293 w303] -> w286
                  tunnel: w287 -> [w295 _]
                  frame No Error {
                    n177 = local read "image pointers 2"() -> (w300:u64[])
                    n178 = Enqueue Element(queue=w295, element=w296, error in (no error)=w294) -> (error out=w293:errorcluster)  [unwired: 1 in, 2 out]
                    n179 = local read "count 2"() -> (w302:i32)
                    n180 = local read "imageNo 2"() -> (w297:i32)
                    n181 = Increment(x=w302) -> (x+1=w301:i32)
                    n182 = Insert Into Array(array=w300, index=w297, new element=w296) -> (w299:u64[])
                    n183 = Increment(x=w297) -> (x+1=w298:i32)
                    n184 = local write "count 2"(w301) -> ()
                    n185 = local write "imageNo 2"(w298) -> ()
                    n186 = local write "image pointers 2"(w299) -> ()
                  }
                  frame Error {
                  }
                }
                n187 = local read "Break"() -> (w285:bool)
              }
            }
            frame #1 {
              n188 = call <userlib>:"AT Command A.vi"("Feature"="AcquisitionStop" ("Command"), "Handle"=w305) -> ()  [unwired: 8 in, 2 out]
            }
            frame #2 {
              n189 = call <userlib>:"AT Flush A.vi"("Handle"=w311) -> ()  [unwired: 9 in, 2 out]
              n190 = call <userlib>:"AT Clear All Buffers A.vi"("Handle"=w311) -> ("error out"=w310:errorcluster)  [unwired: 9 in, 1 out]
              n191 = Merge Errors(w310, w312) -> (w313:errorcluster)
            }
          }
          n192 = Release Queue(queue=w164, error in (no error)=w162) -> (error out=w165:errorcluster)  [unwired: 1 in, 2 out]
          n193 = Merge Errors(w165, w163) -> (w175:errorcluster)
          "error dequeue 2" <- w163
        }
        frame condition #1 {
        }
      }
      n194 = call "SCD - Timestamp AO Waveform.vi"("DAQ To"=w58, "SCD AO Waveforms"=w84) -> ()  [unwired: 8 in, 2 out]
      n195 = Multiply(x=1.25, y=w73) -> (x*y=w108:dbl)
      n196 = call <vilib>:"DAQmx Start Task.vi"("task/channels in"=w52, "error in"=w99) -> ("task out"=w126:refnum<k21>, "error out"=w35:errorcluster)  [unwired: 12 in]
      n197 = call "PDSS - Turn Trigger Light On.vi"("error in (no error)"=w35) -> ("error out"=w115:errorcluster, "Trigger Started"=→"Image Acquisition Started":bool)  [unwired: 9 in]
      n198 = Multiply(x=1000.0, y=w73) -> (x*y=w36:dbl)
      n199 = property on="Image Acq (s)" class="Slide (strict)"(error in=w35, "Scale.Maximum"=w36) -> (error out=w34:errorcluster)  [unwired: 1 in, 1 out]
      n200 = call <vilib>:"DAQmx Wait Until Done.vi"("task/channels in"=w126, "timeout (sec)"=w108, "error in"=w115) -> ("task out"=w125:refnum<k21>, "error out"=w124:errorcluster)  [unwired: 11 in]
      n201 = call <vilib>:"DAQmx Stop Task.vi"("task/channels in"=w125, "error in"=w124) -> ("task out"=w123:refnum<k21>, "error out"=w122:errorcluster)  [unwired: 12 in]
      n202 = call <vilib>:"DAQmx Clear Task.vi"("task in"=w123, "error in"=w122) -> ("error out"=w110:errorcluster)  [unwired: 13 in]
      n203 = while {
        tunnel: w36 -> [w136]
        tunnel: w34 -> [_]
        i -> [w134]
        stop <- w132 stop-if-true
        w133 = u32 100 ("milliseconds to wait")
        n204 = Multiply(x=w134, y=w133) -> (x*y=w137:u32)
        n205 = Wait (ms)(milliseconds to wait=w133) -> ()  [unwired: 1 out]
        n206 = Subtract(x=w136, y=w137) -> (x-y=w130:dbl)
        "Image Acq (s)" <- w130
        n207 = Less Or Equal To 0?(x=w130) -> (x <= 0?=w135:bool)
        n208 = local read "Break"() -> (w131:bool)
        n209 = Or(x=w131, y=w135) -> (x .or. y?=w132:bool)
      }
      n210 = invoke on="Image Acquisition Started" class="Bool (strict)" method="Reinit To Default"(error in=w110) -> (error out=w109:errorcluster)  [unwired: 2 in, 2 out]
      n211 = disable-structure shown="SCMP==SCD" {
        disable-tunnel: [tag "PXI-6733/port0/line0" ("lines") tag "Dev3/port0/line0" ("comp lines")] -> w81
        disable-tunnel: [tag "PXI-6733/ao0:7" ("physical channels") tag "Dev3/ao0:7" ("physical channels")] -> w80
        frame condition #0 {
        }
        frame condition #1 (active) {
        }
      }
      n212 = call "SCD - Trigger Sequence - Set All AO Values to Zero.vi"("error in"=w109, "lines"=w81, "physical channels"=w80) -> ("error out"=w103:errorcluster)  [unwired: 8 in]
      n213 = Release Queue(queue=w22, error in (no error)=w20) -> (error out=w21:errorcluster)  [unwired: 1 in, 2 out]
      n214 = Release Queue(queue=w90, error in (no error)=w89) -> (error out=w83:errorcluster)  [unwired: 1 in, 2 out]
      n215 = Merge Errors(w46, w83, w55, w21) -> (w54:errorcluster)
      n216 = Merge Errors(w54, w103) -> (w102:errorcluster)
      "Headers Out" <- w88
      "error cam dequeue & queue RAM" <- w55
      "Time Start" <- w58
      "error dequeue RAM" <- w20
    }
    frame Error {
    }
  }
  "error out" <- w9
  n217 = disable-structure shown="Disabled" {
    frame Disabled {
      # "someday this\nmight speed up\naccumulatons"
      n218 = call "SCD - Extract Image Vector and Timestamp from Pointer.vi"() -> ()  [unwired: 13 in, 3 out]
    }
    frame Enabled {
    }
  }
